vi "Get Resul Test .vi"(8 "error in (no error)":errorcluster caption="entrée d'erreur (pas d'erreur)", 11 "Class Camera  IV3-500CA - Start Program en entrée":refnum<class "Class Camera  IV3-500CA - Start Program.lvclass">) -> (0 "error out":errorcluster caption="sortie d'erreur", 2 "Resul Test":bool, 3 "Class Camera  IV3-500CA - Start Program en sortie":refnum<class "Class Camera  IV3-500CA - Start Program.lvclass">)   [LabVIEW 2020, in "Library Instrument & Equipement.lvlib" / "Library Camera.lvlib" / "Class Camera  IV3-500CA - Start Program.lvclass"]
uses:
  Class Camera  IV3-500CA - Start Program.lvclass
  Class Camera  IV3-500CA - Start Program.lvclass/Class Camera  IV3-500CA - Start Program.ctl
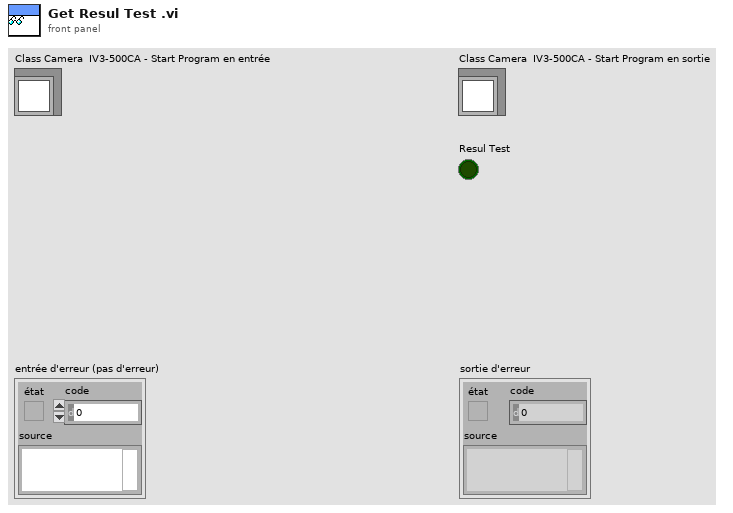
[diagram p1: front panel]
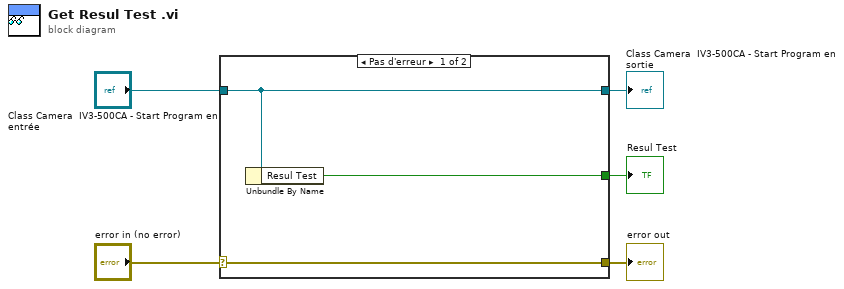
[diagram p0: block diagram]
diagram:
  n1 = case shown="Pas d'erreur" "error in (no error)" {
    selector: "error in (no error)" -> [w8 w9]
    tunnel: [w8 w9] -> w4
    tunnel: [w7 w10] -> w2
    tunnel: "Class Camera  IV3-500CA - Start Program en entrée" -> [w7 w10]
    tunnel: [w6 _] -> w1
    frame No Error {
      n2 = Unbundle By Name(w7) -> ("Resul Test"=w6:bool)
    }
    frame Error {
    }
  }
  "error out" <- w4
  "Class Camera  IV3-500CA - Start Program en sortie" <- w2
  "Resul Test" <- w1
